vi "close.vi"   [LabVIEW 2013]
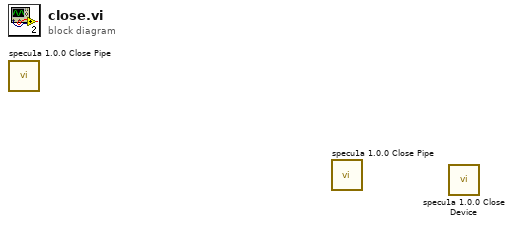
[diagram p0: block diagram]
diagram:
  n1 = call <instrlib>:"specu1a 1.0.0 Close Pipe.vi"() -> ()  [unwired: 4 in, 2 out]
  n2 = call <instrlib>:"specu1a 1.0.0 Close Pipe.vi"() -> ()  [unwired: 4 in, 2 out]
  n3 = call <instrlib>:"specu1a 1.0.0 Close Device.vi"() -> ()  [unwired: 5 in, 1 out]
